vi "Choreo_Choreo_GetTrajectory.vi"(11 "FileName":string="C:\\Users\\Jim\\Desktop\\PathPlanner24\\Choreo\\ChoreoTest.TRAJ") -> (0 "error out":errorcluster, 3 "ChoreoTrajectory":T1, 4 "Full Filename":string)   [LabVIEW 2019, in "ChoreoLib.lvlib"]
doc: "Load a Choreo trajectory from a JSON formatted file. Note that for newer versions of Choreo, the file has a \".traj\" extension. Internally this is formatted as a JSON file.\n\nInputs: \n - filename - string - The name of the trajectory file. See notes below on file naming.\n\nOutputs:\n - Trajectory - cluster - Trajectory read from JSON file.\n - Error out - cluster - Error cluster\n - Full Filename - string - fully qualified file name.\n\nNotes on file naming:\n - The file name must include the extention. \".json\", or \".traj\" is not automatically appended to the name. \n - The file name can be a simple file or an absolute path. If a simple file name is used the default path on the RoboRIO is: \"home:\\lvuser\\natinst\\LabVIEW Data\". On a Windows PC the default path is the LabVIEW default directory. Normally this is: “%HOMEDRIVE%%HOMEPATH%\\Documents\\LabView Data\".\n - Filenames on the RoboRIO, which runs Linux, are case sensitive."
uses:
  ChoreoLib.lvlib
  TypeDef/ChoreoTrajectory.ctl
  TypeDef/ChoreoTrajectoryState.ctl
panel:
  in  "error in (no error)":errorcluster
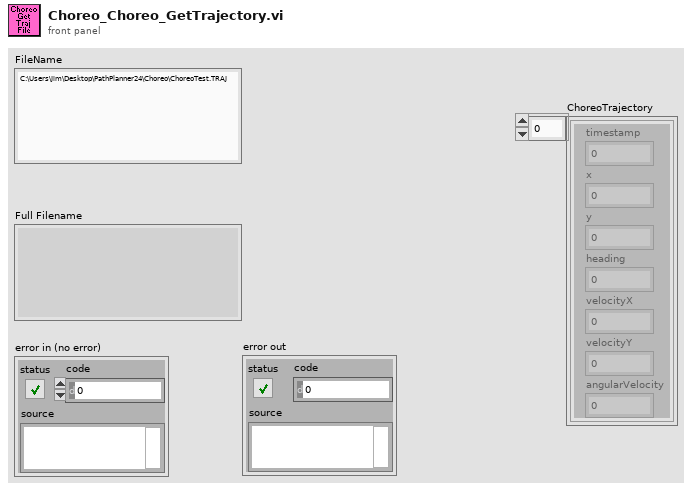
[diagram p1: front panel]
types:
  T1 = typedef "ChoreoLib.lvlib/ChoreoTrajectory.ctl" = T2[]
  T2 = typedef "ChoreoLib.lvlib/ChoreoTrajectoryState.ctl" = cluster{"timestamp":dbl, "x":dbl, "y":dbl, "heading":dbl, "velocityX":dbl, "velocityY":dbl, "angularVelocity":dbl}
  T3 = enum16{"open", "replace", "create", "open or create", "replace or create", "replace or create with confirmation"}
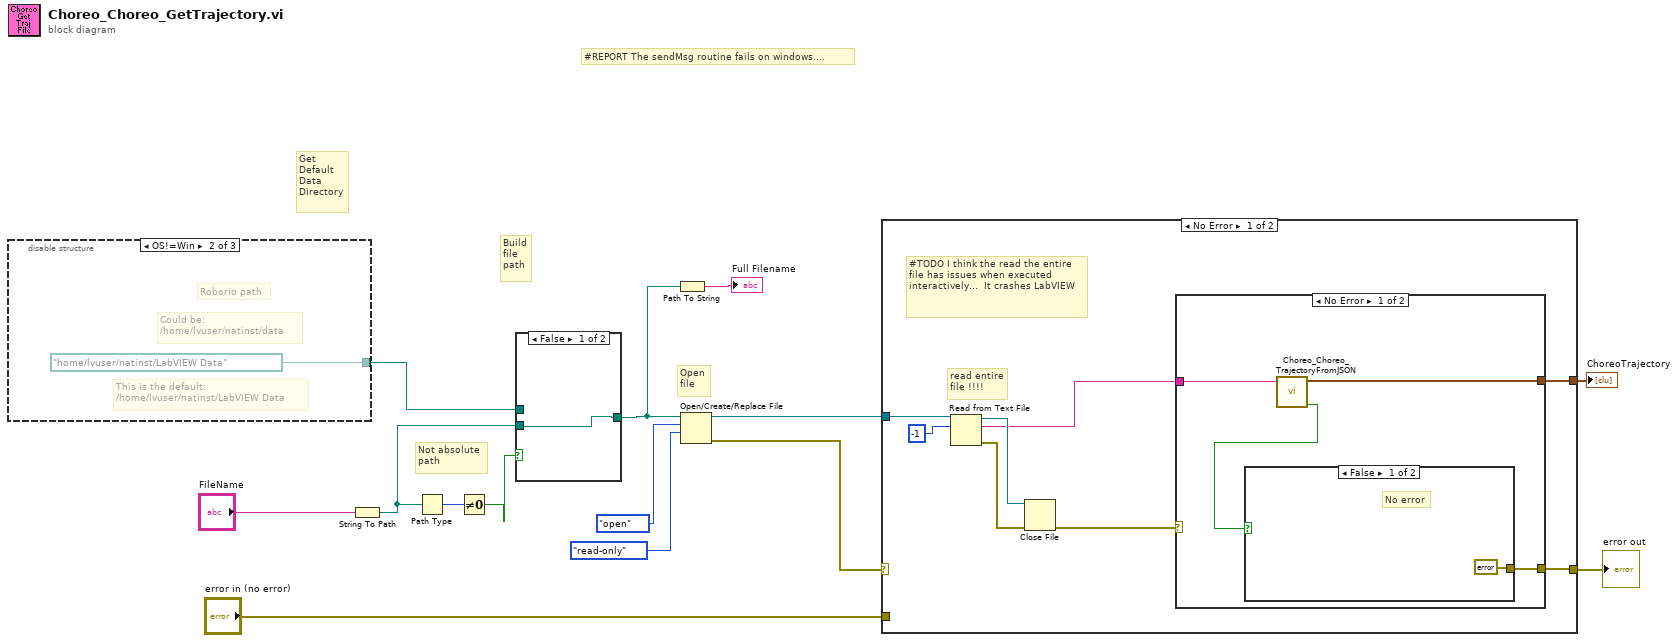
[diagram p0: block diagram]
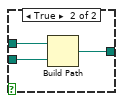
[diagram p2: hidden frame]
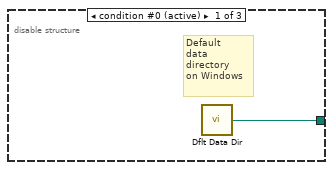
[diagram p3: hidden frame]
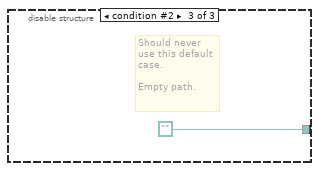
[diagram p4: hidden frame]
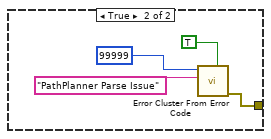
[diagram p5: hidden frame]
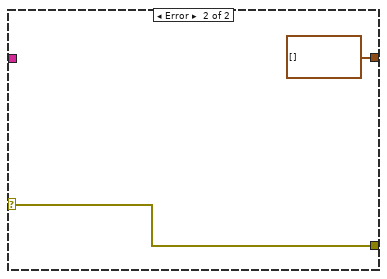
[diagram p6: hidden frame]
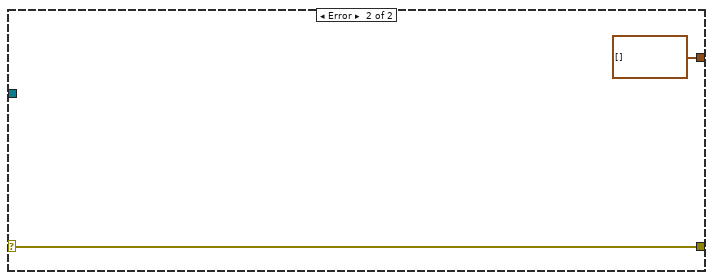
[diagram p7: hidden frame]
diagram:
  # "Not absolute\npath"
  # "#REPORT The sendMsg routine fails on windows...."
  # "Get\nDefault\nData\nDirectory"
  # "Open\nfile"
  # "Build\nfile\npath"
  n1 = disable-structure shown="OS!=Win" {
    disable-tunnel: [w15 path "/home/lvuser/natinst/LabVIEW Data" path ""] -> w11
    frame condition #0 (active) {
      # "Default\ndata\ndirectory\non Windows"
      n2 = call <vilib>:"Dflt Data Dir.vi"() -> ("App:Default Data Directory"=w15:path)
    }
    frame condition #1 {
      # "This is the default:\n/home/lvuser/natinst/LabVIEW Data"
      # "Could be:\n/home/lvuser/natinst/data"
      # "Roborio path"
    }
    frame condition #2 {
      # "Should never\nuse this default\ncase.\n\nEmpty path."
    }
  }
  n3 = String To Path(string="FileName") -> (path=w10:path)
  n4 = Path Type(1:w10) -> (0:w9:i16)
  n5 = Not Equal To 0?(x=w9) -> (x != 0?=w8:bool)
  n6 = case shown="False" w8 {
    tunnel: [w18 w21] -> w5
    tunnel: w11 -> [_ w20]
    tunnel: w10 -> [w18 w19]
    frame False {
    }
    frame True {
      n7 = Build Path(base path=w20, name or relative path=w19) -> (appended path=w21:path)
    }
  }
  n8 = Path To String(path=w5) -> (string=→"Full Filename":string)
  n9 = Open/Create/Replace File(file path (use dialog)=w5, operation (0:open)=T3."open", access (0:read/write)=enum16{"read/write", "read-only", "write-only"}."read-only") -> (refnum out=w6:refnum<file>, error out=w12:errorcluster)  [unwired: 3 in, 1 out]
  n10 = case shown="No Error" w12 {
    selector: w12 -> [_ w42]
    tunnel: w6 -> [w28 _]
    tunnel: [w23 w42] -> w2
    tunnel: "error in (no error)" -> [_ _]
    tunnel: [w22 T1 [] ("ChoreoTrajectory")] -> w1
    frame No Error {
      # "#TODO I think the read the entire\nfile has issues when executed\ninteractively...  It crashes LabVIEW"
      # "read entire\nfile !!!!"
      n11 = Read from Text File(file (use dialog)=w28, count=-1) -> (refnum out=w27:refnum<file>, text=w26:string, error out=w25:errorcluster)  [unwired: 2 in, 1 out]
      n12 = Close File(refnum=w27, error in=w25) -> (error out=w24:errorcluster)  [unwired: 1 out]
      n13 = case shown="No Error" w24 {
        selector: w24 -> [_ w40]
        tunnel: w26 -> [w33 _]
        tunnel: [w31 w40] -> w23
        tunnel: [w30 T1 [] ("ChoreoTrajectory")] -> w22
        frame No Error {
          n14 = call "Choreo_Choreo_TrajectoryFromJSON.vi"("JSON String"=w33) -> ("Error"=w32:bool, "ChoreoTrajectory"=w30:T1)  [unwired: 9 in]
          n15 = case shown="False" w32 {
            tunnel: [errorcluster {"status"=FALSE, "code"=0, "source"=""} ("error out") w35] -> w31
            frame False {
              # "No error"
            }
            frame True {
              n16 = call <vilib>:"Error Cluster From Error Code.vi"("is warning? (False)"=TRUE, "error message (\"\")"="PathPlanner Parse Issue" ("error message (\"\")"), "error code (0)"=99999) -> ("error out"=w35:errorcluster)  [unwired: 6 in]
            }
          }
        }
        frame Error {
        }
      }
    }
    frame Error {
    }
  }
  "error out" <- w2
  "ChoreoTrajectory" <- w1
